vi "Test-SMObase.vi"() -> ()   [LabVIEW 2013]
uses:
  SMO/Typedefs/SMOState --Enum.ctl
  SMO/SMO.lvclass
  Registry/Registry-SMO.lvclass
panel:
  out "Second Pump Qualified Name":string
  out "Registered":string[](array[string])
  out "First Pump Qualified Name":string
  out "Second Pump Instance Name":string
  out "First Pump Instance Name":string
  out "Warning 42 expected":errorcluster
  out "System Name":string
  out "SMO State":T1
  in  "Stop":bool
  out "error out":errorcluster
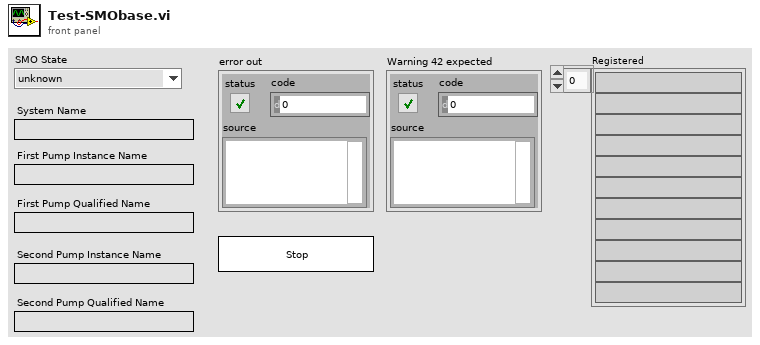
[diagram p1: front panel]
types:
  T1 = typedef "SMO.lvclass/SMOState --Enum.ctl" = enum16{"unknown", "Created", "Started", "Stopped"}
  T2 = typedef "Registry-SMO.lvclass/PublicRegistryEvents--Cluster.ctl" = cluster{"Register Event":refnum<user-event>, "Unregister Event":refnum<user-event>}
  T3 = typedef "SMO.lvclass/Public Events.ctl" = cluster{"Error":refnum<user-event>, "State":refnum<user-event>}
  T4 = cluster{"Event Registration Refnum":refnum<event-registration>}
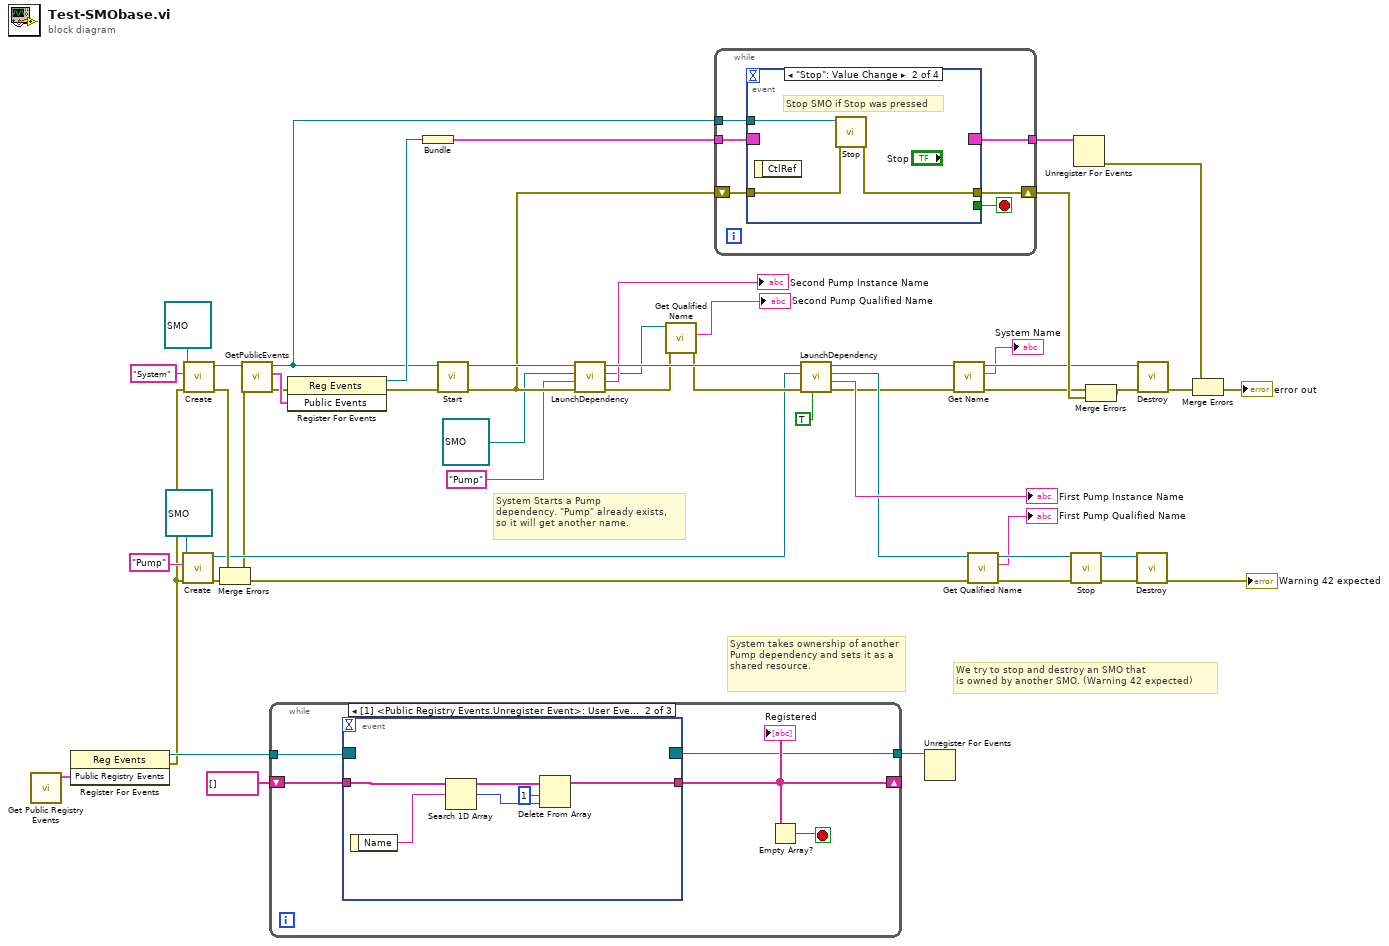
[diagram p0: block diagram]
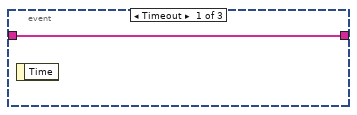
[diagram p2: hidden frame]
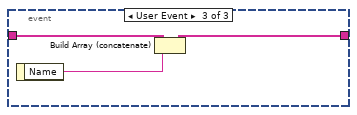
[diagram p3: hidden frame]
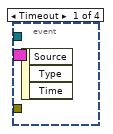
[diagram p4: hidden frame]
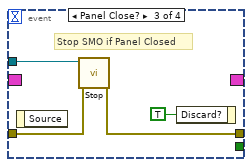
[diagram p5: hidden frame]
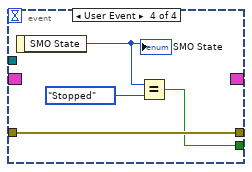
[diagram p6: hidden frame]
diagram:
  # "System Starts a Pump\ndependency. \"Pump\" already exists,\nso it will get another name."
  # "We try to stop and destroy an SMO that\nis owned by another SMO. (Warning 42 expected)"
  # "System takes ownership of another Pump dependency and sets it as a shared resource."
  n1 = call "Get Public Registry Events.vi"() -> ("Public Registry Events"=w14:T2)  [unwired: 10 in, 1 out]
  n2 = register-events(w14) -> (reference out=w13:refnum<event-registration>, error out=w12:errorcluster)  [unwired: 2 in]
  n3 = call "Create.vi"("error in (no error)"=w12, "Subsystem Name (optional)"="Pump", "SMO"=refnum<class "SMO.lvclass"> refnum ("SMO.lvclass")) -> ("error out"=w19:errorcluster, "SMO out"=w6:refnum<class "SMO.lvclass">)  [unwired: 6 in, 1 out]
  n4 = call "Create.vi"("error in (no error)"=w12, "Subsystem Name (optional)"="System", "SMO"=refnum<class "SMO.lvclass"> refnum ("SMO.lvclass")) -> ("error out"=w18:errorcluster, "SMO out"=w42:refnum<class "SMO.lvclass">)  [unwired: 6 in, 1 out]
  n5 = Merge Errors(w18, w19) -> (w2:errorcluster)
  n6 = call "GetPublicEvents.vi"("error in (no error)"=w2, "SMO"=w42) -> ("error out"=w39:errorcluster, "Public Events"=w41:T3, "SMO out"=w40:refnum<class "SMO.lvclass">)  [unwired: 7 in]
  n7 = while {
    tunnel: w13 -> [w55]
    shift-right: [w53] -> _
    shift-left: string[] [] -> [w54]
    tunnel: [w51] -> w10
    stop <- w52 stop-if-true
    n8 = event shown="[1] <Public Registry Events.Unregister Event>: User Event" {
      selector: w55 -> [_ _ _]
      dyn-events: [_ _ _] -> w51
      timeout: _ -> [_ _ _]
      tunnel: w54 -> [w56 w60 w64]
      tunnel: [w56 w59 w62] -> w53
      event Timeout {
        n9 = event-data() -> ()  [unwired: 1 in, 1 out]
      }
      event User Event {
        n10 = event-data() -> ("Name"=w61:string)  [unwired: 1 in]
        n11 = Search 1D Array(1D array=w60, element=w61) -> (index of element=w58:i32)  [unwired: 1 in]
        n12 = Delete From Array(array=w60, length=1, index=w58) -> (array with subset deleted=w59:string[])  [unwired: 1 out]
      }
      event User Event {
        n13 = event-data() -> ("Name"=w63:string)  [unwired: 1 in]
        n14 = Build Array (concatenate)(w64, w63) -> (w62:string[])
      }
    }
    "Registered" <- w53
    n15 = Empty Array?(array=w53) -> (empty?=w52:bool)
  }
  n16 = register-events(error in=w39, w41) -> (reference out=w44:refnum<event-registration>, error out=w43:errorcluster)  [unwired: 1 in]
  n17 = Bundle("Event Registration Refnum"=w44) -> (w49:T4)  [unwired: 1 in]
  n18 = call "Start.vi"("error in (no error)"=w43, "SMO"=w40) -> ("error out"=w23:errorcluster, "SMO out"=w25:refnum<class "SMO.lvclass">)  [unwired: 8 in]
  n19 = call "LaunchDependency.vi"("error in (no error)"=w23, "Dependency Name"="Pump" ("Subsystem Name (optional)"), "Dependency Type"=refnum<class "SMO.lvclass"> refnum ("SMO.lvclass"), "SMO in"=w25) -> ("error out"=w8:errorcluster, "Unique Name"=→"Second Pump Instance Name":string, "Dependency Reference"=w9:refnum<class "SMO.lvclass">, "SMO out"=w24:refnum<class "SMO.lvclass">)  [unwired: 4 in]
  n20 = call "Get Qualified Name.vi"("error in (no error)"=w8, "SMO"=w9) -> ("error out"=w7:errorcluster, "Qualified Name"=→"Second Pump Qualified Name":string)  [unwired: 7 in, 1 out]
  n21 = while {
    shift-right: [w69] -> w48
    shift-left: w23 -> [w68]
    tunnel: w49 -> [w67]
    tunnel: [w66] -> w50
    tunnel: w40 -> [w65]
    stop <- w70 stop-if-true
    n22 = event shown="[1] \"Stop\": Value Change" {
      selector: w67 -> [_ _ _ _]
      dyn-events: [_ _ _ _] -> w66
      timeout: _ -> [_ _ _ _]
      tunnel: [_ _ _ w78] -> w70
      tunnel: w65 -> [_ w73 w77 _]
      tunnel: [_ w72 w76 w79] -> w69
      tunnel: w68 -> [_ w71 w75 w79]
      event Timeout {
        n23 = event-data() -> ()  [unwired: 1 in, 3 out]
      }
      event "Stop": Value Change {
        # "Stop SMO if Stop was pressed"
        n24 = event-data() -> ()  [unwired: 1 in, 1 out]
        n25 = call "Stop.vi"("error in (no error)"=w71, "SMO"=w73) -> ("error out"=w72:errorcluster)  [unwired: 8 in, 1 out]
      }
      event Panel Close? {
        # "Stop SMO if Panel Closed"
        n26 = event-data() -> ()  [unwired: 1 in, 1 out]
        n27 = call "Stop.vi"("error in (no error)"=w75, "SMO"=w77) -> ("error out"=w76:errorcluster)  [unwired: 8 in, 1 out]
        n28 = event-data("Discard?"=TRUE ("OK")) -> ()  [unwired: 1 in, 1 out]
      }
      event User Event {
        n29 = event-data() -> ("SMO State"=w81:T1)  [unwired: 1 in]
        "SMO State" <- w81
        n30 = Equal?(x=w81, y=SMOState_--Enum."Stopped") -> (x = y?=w78:bool)
      }
    }
  }
  n31 = call "LaunchDependency.vi"("Shared Resource"=TRUE, "error in (no error)"=w7, "Dependency Type"=w6, "SMO in"=w24) -> ("error out"=w3:errorcluster, "Unique Name"=→"First Pump Instance Name":string, "Dependency Reference"=w5:refnum<class "SMO.lvclass">, "SMO out"=w4:refnum<class "SMO.lvclass">)  [unwired: 4 in]
  n32 = Unregister For Events(event registration refnum=w10) -> ()  [unwired: 1 in, 1 out]
  n33 = call "Get Name.vi"("error in (no error)"=w3, "SMO"=w4) -> ("error out"=w36:errorcluster, "Name"=→"System Name":string, "SMO out"=w37:refnum<class "SMO.lvclass">)  [unwired: 7 in]
  n34 = call "Get Qualified Name.vi"("error in (no error)"=w2, "SMO"=w5) -> ("error out"=w16:errorcluster, "Qualified Name"=→"First Pump Qualified Name":string, "SMO out"=w17:refnum<class "SMO.lvclass">)  [unwired: 7 in]
  n35 = call "Stop.vi"("error in (no error)"=w16, "SMO"=w17) -> ("error out"=w31:errorcluster, "SMO out"=w32:refnum<class "SMO.lvclass">)  [unwired: 8 in]
  n36 = Unregister For Events(event registration refnum=w50) -> (error out=w47:errorcluster)  [unwired: 1 in]
  n37 = Merge Errors(w36, w48) -> (w38:errorcluster)
  n38 = call "Destroy.vi"("error in (no error)"=w31, "SMO"=w32) -> ("error out"=→"Warning 42 expected":errorcluster)  [unwired: 9 in]
  n39 = call "Destroy.vi"("error in (no error)"=w38, "SMO"=w37) -> ("error out"=w45:errorcluster)  [unwired: 9 in]
  n40 = Merge Errors(w47, w45) -> (→"error out":errorcluster)
